vi "WPI_CameraGet Exposure.vi"(8 "error in (no error)":errorcluster, 11 "CameraDevRef":T1={"Camera Address"="192.168.0.90", "CameraStatus"={"status"=FALSE, "code"=0, "source"=""}}) -> (0 "error out":errorcluster, 1 "Exposure (%)":dbl, 2 "Exposure":T2, 3 "CameraDevRef Out":T1)   [LabVIEW 2017]
doc: "Returns the exposure setting of the camera you specify.\n\nThis software is licensed. Open the labview\\readme\\WPI Robotics Library Open Source License.txt file for more information."
uses:
  <vilib>/Rock Robotics/WPI/Camera/WPI_CameraExposure Values.ctl
  <vilib>/Rock Robotics/WPI/Camera/WPI_CameraDevRef.ctl
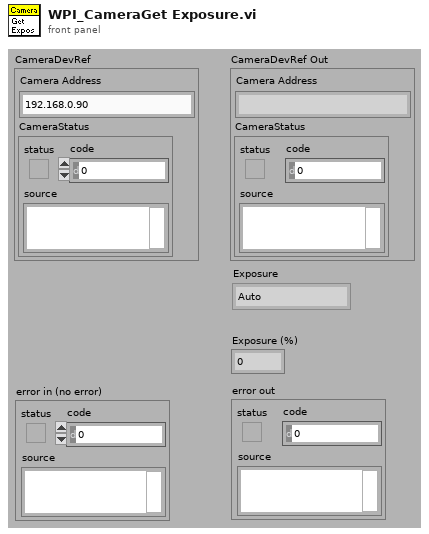
[diagram p1: front panel]
types:
  T1 = typedef "WPI_CameraDevRef.ctl" = cluster{"Camera Address":string, "CameraStatus":errorcluster}
  T2 = typedef "WPI_CameraExposure Values.ctl" = enum16{"Auto", "Flicker-free 50 Hz", "Flicker-free 60 Hz", "Hold current", "Custom"}
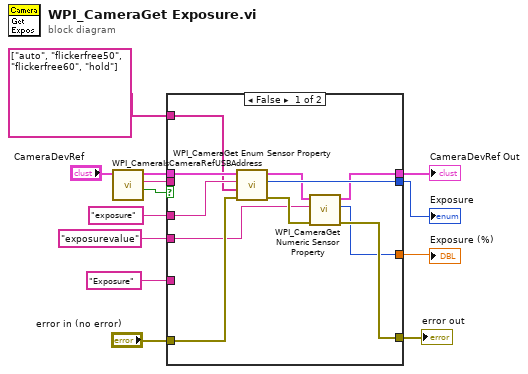
[diagram p0: block diagram]
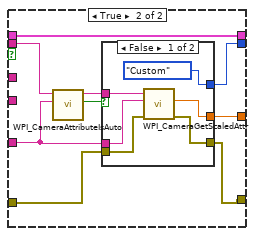
[diagram p2: hidden frame]
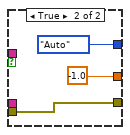
[diagram p3: hidden frame]
diagram:
  n1 = call <vilib>:"WPI_CameraIsCameraRefUSBAddress.vi"("CameraDevRef"="CameraDevRef") -> ("USB?"=w4:bool, "Camera Address Out"=w5:string, "CameraDevRef out"=w2:T1)  [unwired: 7 in, 1 out]
  n2 = case shown="False" w4 {
    tunnel: "exposure" ("format string") -> [w24 _]
    tunnel: "error in (no error)" -> [w23 w26]
    tunnel: [w22 w27] -> w11
    tunnel: [w19 w29] -> w10
    tunnel: [w17 w25] -> w9
    tunnel: w2 -> [w21 w29]
    tunnel: w5 -> [_ w30]
    tunnel: "Exposure" -> [_ w31]
    tunnel: [w15 w28] -> w7
    tunnel: "exposurevalue" ("format string") -> [w16 _]
    tunnel: string[] ["auto", "flickerfree50", "flickerfree60", "hold"] -> [w14 _]
    frame False {
      n3 = call <vilib>:"WPI_CameraGet Enum Sensor Property.vi"("error in (no error)"=w23, "Strings"=w14, "Property Name"=w24, "CameraDevRef"=w21) -> ("error out"=w18:errorcluster, "Enum Int Value"=w22:i32, "CameraDevRef out"=w20:T1)  [unwired: 2 in, 3 out]
      n4 = call <vilib>:"WPI_CameraGet Numeric Sensor Property.vi"("error in (no error)"=w18, "Property Name"=w16, "CameraDevRef"=w20) -> ("error out"=w17:errorcluster, "Value"=w15:i32, "CameraDevRef dup"=w19:T1)  [unwired: 6 in]
    }
    frame True {
      n5 = call <vilib>:"WPI_CameraAttributeIsAuto.vi"("Attr String"=w31, "Camera Address In"=w30) -> ("Auto?"=w33:bool, "Camera Address Out"=w32:string)  [unwired: 8 in]
      n6 = case shown="False" w33 {
        tunnel: w31 -> [w38 _]
        tunnel: w32 -> [w39 _]
        tunnel: [w34 -1.0] -> w28
        tunnel: [WPI_CameraExposure_Values."Custom" ("Exposure") WPI_CameraExposure_Values."Auto" ("Exposure")] -> w27
        tunnel: [w36 w40] -> w25
        tunnel: w26 -> [w35 w40]
        frame False {
          n7 = call <vilib>:"WPI_CameraGetScaledAttr.vi"("error in (no error)"=w35, "Attr String"=w38, "Camera Address In"=w39) -> ("error out"=w36:errorcluster, "Scaled"=w34:dbl)  [unwired: 5 in, 2 out]
        }
        frame True {
        }
      }
    }
  }
  "Exposure" <- w11
  "CameraDevRef Out" <- w10
  "error out" <- w9
  "Exposure (%)" <- w7
